vi "F_Update_B.vi"(8 "错误输入（无错误）":errorcluster, 11 "引用":refnum<k24>) -> (0 "错误输出":errorcluster, 1 "*.license文件路径":path, 2 "F_Update_B":bool, 3 "引用输出":refnum<k24>)   [LabVIEW 2013]
uses:
  AuthorizationToolClassLibrary.dll
panel:
  out "P_ErroInfo_S":string
  # "是否升级成功"
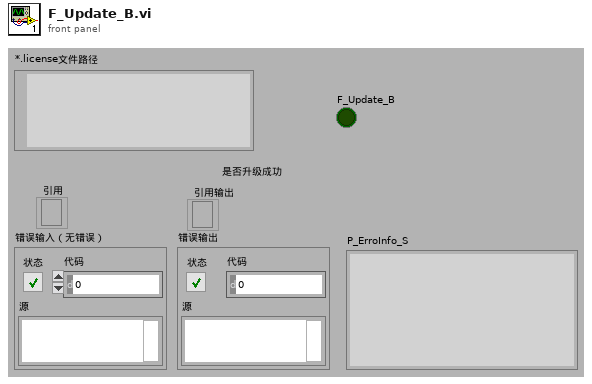
[diagram p1: front panel]
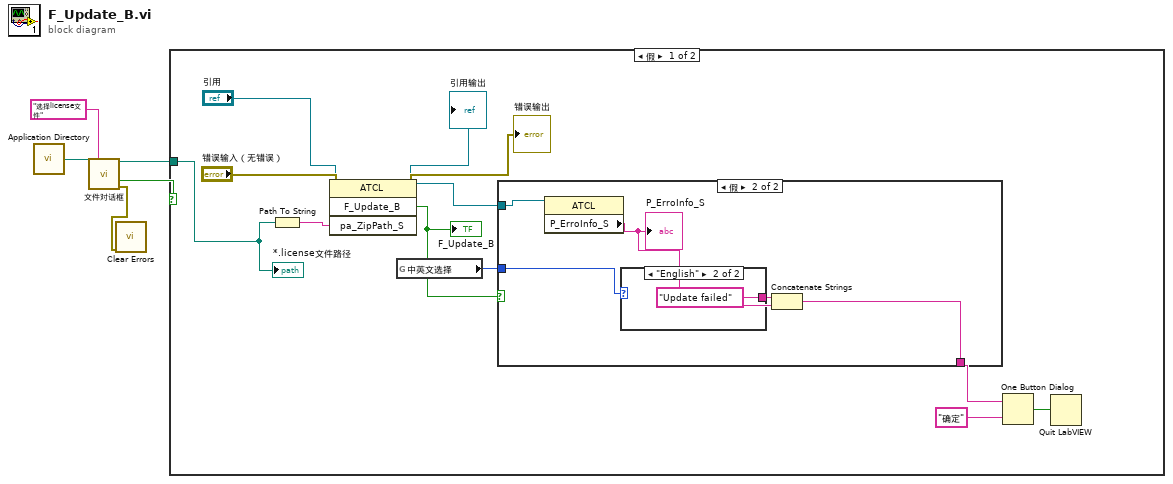
[diagram p0: block diagram]
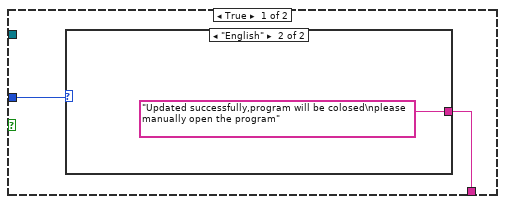
[diagram p2: hidden frame]
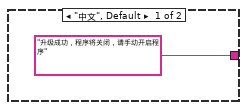
[diagram p3: hidden frame]
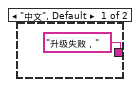
[diagram p4: hidden frame]
diagram:
  n1 = call <vilib>:"Application Directory.vi"() -> ("Application Directory"=w3:path)
  n2 = call "文件对话框"("start path"=w3, "prompt"="选择license文件") -> ("selected path"=w4:path, "cancelled"=w5:bool, "error out"=w1:errorcluster)  [unwired: 10 in, 1 out]
  n3 = call <vilib>:"Clear Errors.vi"("error in (no error)"=w1) -> ()  [unwired: 6 in, 1 out]
  n4 = case shown="假" w5 {
    tunnel: w4 -> [w15 _]
    frame False {
      n5 = Path To String(path=w15) -> (string=w10:string)
      n6 = invoke class="ATCL" method="F_Update_B"(reference="引用", error in="错误输入（无错误）", "pa_ZipPath_S"=w10) -> (reference out=w8:refnum<k24>, error out=→"错误输出":errorcluster, "F_Update_B"=w11:bool)  [unwired: 1 in, 1 out]
      "F_Update_B" <- w11
      "引用输出" <- w8
      n7 = global read "中英文全局.vi" "中英文选择"() -> (w7:enum32{"中文", "English"})
      n8 = case shown="假" w11 {
        tunnel: [w18 w22] -> w12
        tunnel: w8 -> [_ w25]
        tunnel: w7 -> [w17 w21]
        frame True {
          n9 = case shown="\"English\"" w17 {
            tunnel: ["升级成功，程序将关闭，请手动开启程序" ("搜索字符串/字符(-)") "Updated successfully,program will be colosed\nplease manually open the program" ("搜索字符串/字符(-)")] -> w18
            frame "中文", Default {
            }
            frame "English" {
            }
          }
        }
        frame False {
          n10 = property class="ATCL"(reference=w25) -> ("P_ErroInfo_S"=w23:string)  [unwired: 1 in, 2 out]
          "P_ErroInfo_S" <- w23
          n11 = case shown="\"English\"" w21 {
            tunnel: ["升级失败，" ("搜索字符串/字符(-)") "Update failed" ("搜索字符串/字符(-)")] -> w24
            frame "中文", Default {
            }
            frame "English" {
            }
          }
          n12 = Concatenate Strings(w24, w23) -> (w22:string)
        }
      }
      n13 = One Button Dialog(message=w12, button name ("OK")="确定" ("按钮名称（“确定”）")) -> (true=w14:bool)
      n14 = Quit LabVIEW(quit? (T)=w14) -> ()
      "*.license文件路径" <- w15
    }
    frame True {
    }
  }
